vi "h5_open_file.vi"(8 "error in":errorcluster, 11 "path (open)":path) -> (0 "error out":errorcluster, 2 "ok?":bool, 3 "h5 root ref":T1 format="%.0x")   [LabVIEW 2015]
uses:
  <vilib>/addons/h5labview2/base/hid_t.ctl
  <vilib>/addons/h5labview2/file/H5Fmode.ctl
  polys/poly_h5_tools_eco_plus.vi
  <vilib>/addons/h5labview2/file/H5F.lvlib
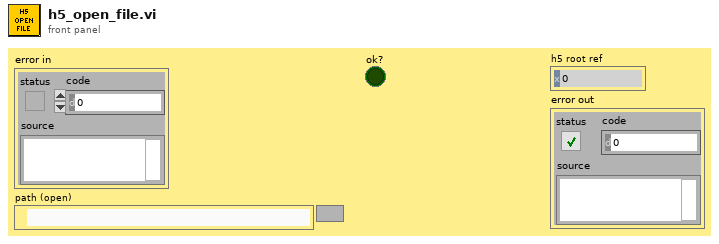
[diagram p1: front panel]
types:
  T1 = typedef "hid_t.ctl" = i32
  T2 = typedef "H5F.lvlib/H5Fmode.ctl" = enum16{"read-only", "read-write", "overwrite", "create new", "open or create"}
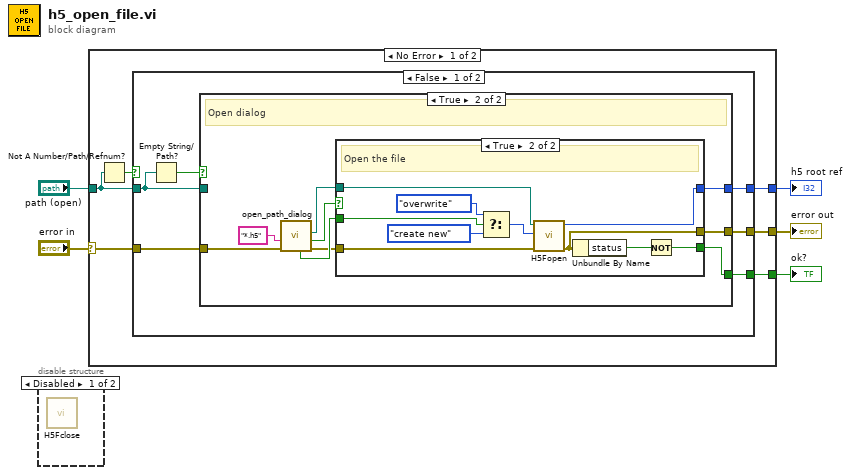
[diagram p0: block diagram]
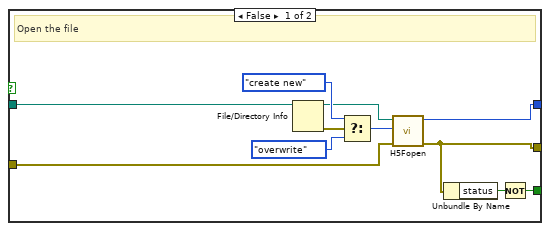
[diagram p3: hidden frame]
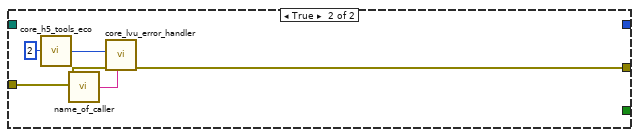
[diagram p5: hidden frame]
diagram:
  n1 = disable-structure shown="Disabled" {
    frame Disabled {
      n2 = call <vilib>:"H5Fclose.vi"() -> ()  [unwired: 11 in, 1 out]
    }
    frame Enabled {
    }
  }
  n3 = case shown="No Error" "error in" {
    selector: "error in" -> [w11 w55]
    tunnel: "path (open)" -> [w10 _]
    tunnel: [w7 w55] -> w2
    tunnel: [w8 _] -> w3
    tunnel: [w6 _] -> w1
    frame No Error {
      n4 = Not A Number/Path/Refnum?(number/path/refnum=w10) -> (NaN/Path/Refnum?=w9:bool)
      n5 = case shown="False" w9 {
        tunnel: w10 -> [w17 _]
        tunnel: w11 -> [w15 w52]
        tunnel: [w13 w50] -> w7
        tunnel: [w12 _] -> w8
        tunnel: [w14 _] -> w6
        frame False {
          n6 = Empty String/Path?(string/path=w17) -> (empty?=w16:bool)
          n7 = case shown="True" w16 {
            tunnel: w17 -> [w25 _]
            tunnel: w15 -> [w22 w36]
            tunnel: [w21 w31] -> w13
            tunnel: [w19 w30] -> w14
            tunnel: [w18 w29] -> w12
            frame False {
              # "Open the file"
              n8 = File/Directory Info(path=w25) -> (path out=w24:path, error out=w28:errorcluster)  [unwired: 1 in, 5 out]
              n9 = Select(t=H5Fmode."create new" ("mode (read-only)"), s=w28, f=H5Fmode."overwrite" ("mode (read-only)")) -> (s? t:f=w23:T2)
              n10 = call <vilib>:"H5Fopen.vi"("error in (no error)"=w22, "mode (read-only)"=w23, "path"=w24) -> ("error out"=w21:errorcluster, "ref out"=w18:T1)  [unwired: 7 in]
              n11 = Unbundle By Name(w21) -> ("status"=w20:bool)
              n12 = Not(x=w20) -> (.not. x?=w19:bool)
            }
            frame True {
              # "Open dialog"
              n13 = call "open_path_dialog.vi"("error in"=w36, "pattern (all files)"="*.h5") -> ("error out"=w32:errorcluster, "ok?"=w35:bool, "path"=w33:path, "exists?"=w34:bool)  [unwired: 6 in]
              n14 = case shown="True" w35 {
                selector: w35 -> [w38 _]
                tunnel: w34 -> [_ w49]
                tunnel: w33 -> [_ w45]
                tunnel: w32 -> [w39 w44]
                tunnel: [w39 w43] -> w31
                tunnel: [w38 w41] -> w30
                tunnel: [_ w40] -> w29
                frame False {
                  # "Do not open a file"
                }
                frame True {
                  # "Open the file"
                  n15 = Select(t=H5Fmode."overwrite" ("mode (read-only)"), s=w49, f=H5Fmode."create new" ("mode (read-only)")) -> (s? t:f=w46:T2)
                  n16 = call <vilib>:"H5Fopen.vi"("error in (no error)"=w44, "mode (read-only)"=w46, "path"=w45) -> ("error out"=w43:errorcluster, "ref out"=w40:T1)  [unwired: 7 in]
                  n17 = Unbundle By Name(w43) -> ("status"=w42:bool)
                  n18 = Not(x=w42) -> (.not. x?=w41:bool)
                }
              }
            }
          }
        }
        frame True {
          n19 = call-poly "core_h5_tools_eco.vi"("code (w/out eco)"=2) -> ("code (+ eco)"=w53:i32)  [unwired: 4 in]
          n20 = call "name_of_caller.vi"() -> ("name of caller out"=w51:string)  [unwired: 4 in]
          n21 = call "core_lvu_error_handler.vi"("name of caller in (you)"=w51, "error in (no error)"=w52, "code (0 = no error)"=w53) -> ("error out"=w50:errorcluster)  [unwired: 7 in, 1 out]
        }
      }
    }
    frame Error {
    }
  }
  "h5 root ref" <- w3
  "error out" <- w2
  "ok?" <- w1
